vi "Main.vi"() -> ()   [LabVIEW 2013] (continued)
                # "Selection Order No"
                n1184 = Concatenate Strings(".*_" ("string"), w1862, "_" ("string")) -> (w1860:string)
              }
            }
            n1185 = call "Folder - Subtract Number of Months.vi"("- # of Months"=0, "YYYYmm"="201301", "Folder"=w1812) -> (">= Range (Folder\\YYYY\\mm)"=w1810:path[])  [unwired: 6 in, 2 out]
            n1186 = for {
              tunnel: [w1828] -> w1809 mode=concatenating
              tunnel: w1810 -> [w1827] mode=indexing
              n1187 = List Folder(path=w1827) -> (filenames=w1828:string[])  [unwired: 3 in, 3 out]
            }
            n1188 = for {
              tunnel: w1823 -> [w1852] mode=indexing
              tunnel: w1822 -> [w1854]
              tunnel: [w1853] -> w1821 mode=indexing
              n1189 = Concatenate Strings(w1854, w1852) -> (w1853:string)
            }
            n1190 = for {
              tunnel: w1821 -> [w1841] mode=indexing
              tunnel: w1809 -> [w1840]
              shift-right: [w1839] -> w1819
              shift-left: string[] [] -> [w1838]
              n1191 = for {
                tunnel: w1841 -> [w1843]
                tunnel: w1840 -> [w1844] mode=indexing
                shift-right: [w1846] -> w1839
                shift-left: w1838 -> [w1845]
                n1192 = Match Pattern(string=w1844, regular expression=w1843) -> (offset past match=w1842:i32)  [unwired: 1 in, 3 out]
                n1193 = Greater Or Equal To 0?(x=w1842) -> (x >= 0?=w1847:bool)
                n1194 = case shown="True" w1847 {
                  tunnel: w1844 -> [_ w1849]
                  tunnel: [w1848 w1851] -> w1846
                  tunnel: w1845 -> [w1848 w1850]
                  frame False {
                  }
                  frame True {
                    n1195 = Build Array (concatenate)(w1850, w1849) -> (w1851:string[])
                  }
                }
              }
            }
            "List Of Files From Selected Reports" <- w1819
            n1196 = for {
              tunnel: w1819 -> [w1837] mode=indexing
              tunnel: [w1836] -> w1818 mode=indexing
              tunnel: [w1833] -> w1817 mode=indexing
              tunnel: [w1829] -> w1814 mode=indexing
              w1834 = "_" ("regular expression")
              n1197 = Match Pattern(string=w1837, regular expression=w1834) -> (before substring=w1836:string, after substring=w1835:string)  [unwired: 1 in, 2 out]
              n1198 = Match Pattern(string=w1835, regular expression=w1834) -> (before substring=w1833:string, after substring=w1832:string)  [unwired: 1 in, 2 out]
              n1199 = Match Pattern(string=w1832, regular expression="\\.") -> (before substring=w1830:string)  [unwired: 1 in, 3 out]
              n1200 = call "String - Convert String Only TimeStamp.vi"("YYYYmmdd_HHMMSS"=w1830) -> ("YYYY-mm-dd HH:MM:SS"=w1829:string)  [unwired: 10 in]
            }
            n1201 = Build Array(w1814, w1818, w1817) -> (w1816:string[][])
            n1202 = Transpose 2D Array(2D array=w1816) -> (transposed array=w1815:string[][])
            n1203 = property on="Report List" class="MCListbox (strict)"("ItemNames"=w1815, "TopLeft"=T34 {"Row"=0, "Column"=0} ("Top Left Visible Cell"), "Value"=-1 ("Report List")) -> ()  [unwired: 2 in, 2 out]
          }
          frame True {
            w1874 = 86400.0  # 60s x 60min x 24hr
            w1879 = "[CreatedOn] >= '<A>' AND [CreatedOn] <= '<B>'"  # AND <AND_CONDITION>
            # "Move to Top"
            # "To cater for Time stored in DB but ignored in Date Control\ni.e. 2014/10/04 13:00 will be 2014/10/04 without the time\nby added 1day, it will now be 2014/10/05 which will take care of\nany TIME during the day of 2014/10/04 stored in DB"
            # "Use DB"
            n1204 = String Length(string=w1889) -> (length=w1891:i32)
            n1205 = Greater Than 0?(x=w1891) -> (x > 0?=w1890:bool)
            n1206 = case shown="True" w1890 {
              tunnel: w1889 -> [w1893 _]
              tunnel: [w1892 w1896] -> w1888
              tunnel: w1887 -> [_ w1895]
              frame True {
                # "Select by TransactionNo"
                n1207 = Bundle("TransactionNo", "Selection Transaction No"=w1893) -> (w1892:cluster{string, "Selection Transaction No":T5})  [unwired: 1 in]
              }
              frame False {
                # "Select by OrderNo"
                n1208 = Bundle("OrderNo", "Selection Order No"=w1895) -> (w1896:cluster{string, "Selection Order No":T5})  [unwired: 1 in]
              }
            }
            n1209 = property on="Date End" class="AbsTime (strict)"() -> ("Value"=w1875:timestamp)  [unwired: 2 in, 2 out]
            n1210 = property on="Date Start" class="AbsTime (strict)"() -> ("Value"=w1877:timestamp)  [unwired: 2 in, 2 out]
            n1211 = global read "Global SRTRS.vi" "Date Format"() -> (w1878:string)
            n1212 = Add(x=w1875, y=w1874) -> (x+y=w1873:timestamp)
            n1213 = Format Date/Time String(time format string (%c)=w1878, seconds (now)=w1877) -> (date/time string=w1883:string)  [unwired: 1 in]
            n1214 = Format Date/Time String(time format string (%c)=w1878, seconds (now)=w1873) -> (date/time string=w1884:string)  [unwired: 1 in]
            n1215 = Search and Replace String(input string=w1879, search string="<A>", replace string=w1883) -> (result string=w1881:string)  [unwired: 5 in, 3 out]
            n1216 = Search and Replace String(input string=w1881, search string="<B>", replace string=w1884) -> (result string=w1876:string)  [unwired: 5 in, 3 out]
            n1217 = call "DB - [Execute].[ReportList].vi"(2:DB_-_Execute_ReportList_Enum."SELECT [TransactionNo],* OR [OrderNo],*", "AND <AND_CONDITION>"=w1876, "Search Cluster"=w1888) -> ("data"=w1872:string[][], "SUMMARY"=w1885:errorcluster)  [unwired: 9 in, 2 out]
            n1218 = local write "DB"(w1885) -> ()
            n1219 = property on="Report List" class="MCListbox (strict)"("ItemNames"=w1872, "TopLeft"=T34 {"Row"=0, "Column"=0} ("Top Left Visible Cell")) -> ()  [unwired: 2 in, 2 out]
            n1220 = Array Size(array=w1872) -> (size(s)=w1871:i32[])
            n1221 = Index Array(array=w1871, index=0) -> (element=w1869:i32)
            n1222 = Greater Than 0?(x=w1869) -> (x > 0?=w1868:bool)
            n1223 = Select(t=T30."Enabled" ("Disabled"), s=w1868, f=T30."Disabled and Grayed Out" ("Disabled")) -> (s? t:f=w1866:T30)
            n1224 = property on="Report Open" class="Bool"("DisabledEnum"=w1866) -> ()  [unwired: 2 in, 2 out]
          }
        }
      }
      event "Report List": Mouse Up {
        # "Mouse UP has best result for sorting Col"
        n1225 = event-data() -> ("CtlRef"=w1900:refnum<vi>)  [unwired: 1 in, 7 out]
        n1226 = control-ref of="Sort Order"() -> (w1899:refnum<vi>)
        n1227 = call "MCListbox Event - Sort Table.vi"("Clicked Color"=u32 16777216, "Sort Order Boolean Ref"=w1899, "MCListBox Ref"=w1900) -> ()  [unwired: 8 in, 1 out]
      }
      event Value Change {
        n1228 = event-data() -> ()  [unwired: 1 in, 6 out]
        n1229 = local read "DB - Report"() -> (w1901:bool)
        n1230 = case shown="True" w1901 {
          frame False {
          }
          frame True {
            n1231 = property on="Selection Order No" class="CmbBox (strict)"() -> ("Value"=w1907:T5)  [unwired: 2 in, 2 out]
            n1232 = property on="Selection Transaction No" class="CmbBox (strict)"() -> ("Value"=w1908:T5)  [unwired: 2 in, 2 out]
            n1233 = call <vilib>:"Trim Whitespace.vi"("string"=w1907) -> ("trimmed string"=w1905:string)  [unwired: 1 in]
            n1234 = call <vilib>:"Trim Whitespace.vi"("string"=w1908) -> ("trimmed string"=w1906:string)  [unwired: 1 in]
            n1235 = String Length(string=w1905) -> (length=w1903:i32)
            n1236 = String Length(string=w1906) -> (length=w1904:i32)
            n1237 = Add(x=w1904, y=w1903) -> (x+y=w1902:i32)
            n1238 = disable-structure shown="Disabled" {
              disable-tunnel: w1902 -> [w1913 _]
              frame Disabled {
                n1239 = Greater Than 0?(x=w1913) -> (x > 0?=w1912:bool)
                n1240 = Select(t=T30."Enabled" ("Disabled"), s=w1912, f=T30."Disabled and Grayed Out" ("Disabled")) -> (s? t:f=w1909:T30)
                n1241 = property on="Report Execute Search" class="Bool"("DisabledEnum"=w1909) -> ()  [unwired: 2 in, 2 out]
              }
              frame Enabled {
              }
            }
          }
        }
      }
      event "FTP File List": Mouse Up {
        # "Mouse Up seems to work BEST for Sorting"
        n1242 = event-data() -> ("CtlRef"=w1914:refnum<vi>)  [unwired: 1 in, 7 out]
        n1243 = control-ref of="Ascending"() -> (w1915:refnum<vi>)
        n1244 = call "MCListbox Event - Sort Table.vi"("Clicked Color"=u32 16777216, "Sort Order Boolean Ref"=w1915, "MCListBox Ref"=w1914) -> ()  [unwired: 8 in, 1 out]
      }
      event "FTP File List": Value Change {
        n1245 = event-data() -> ("NewVal"=w1919:i32)  [unwired: 1 in, 5 out]
        n1246 = global read "Global SRTRS.vi" "[RawDataReport]"() -> (w1917:bool)
        n1247 = Greater Or Equal To 0?(x=w1919) -> (x >= 0?=w1918:bool)
        n1248 = case shown="True" w1917 {
          tunnel: w1918 -> [_ w1923]
          frame False {
          }
          frame True {
            n1249 = Select(t=T30."Enabled" ("Disabled"), s=w1923, f=T30."Disabled and Grayed Out" ("Disabled")) -> (s? t:f=w1922:T30)
            n1250 = property on="cRIO FTP Copy" class="Bool"("DisabledEnum"=w1922) -> ()  [unwired: 2 in, 2 out]
          }
        }
      }
      event "cRIO  Search": Value Change {
        (unwired) "c:\\ni-rt\\LabVIEW Data\\SRTRS4070\\Data\\"
        w1939 = "\\" ("string")
        # "c:\\ni-rt\\LabVIEW Data\\SRTRS4070\\Data\\2014\\04\\"
        # "FTP to cRIO to look for raw data files"
        n1251 = event-data() -> ()  [unwired: 1 in, 6 out]
        n1252 = local read "cRIO IP"() -> (w1946:string)
        n1253 = Format Into String(format string="%02d", "FTP Month") -> (resulting string=w1936:string)  [unwired: 2 in, 1 out]
        n1254 = Format Into String("FTP Year") -> (resulting string=w1940:string)  [unwired: 3 in, 1 out]
        n1255 = Concatenate Strings("u:\\ni-rt\\LabVIEW Data\\SRTRS4070\\Data\\", w1940, w1939, w1936, w1939) -> (w1938:string)
        n1256 = call "cRIO - FTP Module.vi"("List"=TRUE, "Copy"=FALSE, "Source Folder (on RT target)"=w1938, "IP address of remote RT target"=w1946) -> ("Error Out"=w1935:errorcluster, "Files in cRIO"=w1943:string[])  [unwired: 4 in, 2 out]
        n1257 = case shown="No Error" w1935 {
          tunnel: w1943 -> [w1956 _]
          tunnel: [w1951 _] -> w1931
          frame No Error {
            n1258 = String To Path(string=w1956) -> (path=w1955:path[])
            n1259 = for {
              tunnel: w1955 -> [w1964] mode=indexing
              tunnel: [w1958] -> w1954 mode=indexing
              tunnel: [w1957] -> w1953 mode=indexing
              n1260 = Strip Path(path=w1964) -> (name=w1963:string)  [unwired: 1 out]
              n1261 = Match Pattern "Transaction No."(string=w1963, regular expression="_") -> (before substring=w1957:string, after substring=w1962:string)  [unwired: 1 in, 2 out]
              n1262 = Match Pattern "Time Stamp"(string=w1962, regular expression=".dat") -> (before substring=w1959:string)  [unwired: 1 in, 3 out]
              n1263 = call "String - Convert String Only TimeStamp.vi"("YYYYmmdd_HHMMSS"=w1959) -> ("YYYY-mm-dd HH:MM:SS"=w1958:string)  [unwired: 10 in]
            }
            n1264 = Build Array(w1954, w1953) -> (w1952:string[][])
            n1265 = Transpose 2D Array(2D array=w1952) -> (transposed array=w1951:string[][])
            "Files in cRIO" <- w1956
          }
          frame Error {
          }
        }
        n1266 = Array Size(array=w1931) -> (size(s)=w1930:i32[])
        n1267 = Index Array(array=w1930) -> (element=w1924:i32)  [unwired: 1 in]
        n1268 = property on="FTP File List" class="MCListbox (strict)"("ItemNames"=w1931, "TopLeft"=T34 {"Row"=0, "Column"=0} ("Top Left Visible Cell"), "Value"=-1 ("Report List")) -> ()  [unwired: 2 in, 2 out]
        n1269 = Format Into String(w1924) -> (resulting string=w1929:string)  [unwired: 3 in, 1 out]
        n1270 = case shown="0" w1924 {
          frame 1, Default {
          }
          frame 0 {
            n1271 = call "Msgbox - Message Handler.vi"("Short Description (When DB Not Available)"="Raw Data Not Found", "Description (When DB Not Available)"="No raw data files for the given criteria", "<.?....> Message Code"="<E 403>") -> ("MHandler Error"=w1947:errorcluster)  [unwired: 6 in, 2 out]
            n1272 = local write "MHandler"(w1947) -> ()
          }
        }
        n1273 = Concatenate Strings("{cRIO Search} " ("string"), w1929, " file(s) found." ("string")) -> (w1925:string)
        n1274 = call "Queue - EnQueue to MessageQ.vi"("<NoD> Don't Display to UI"=TRUE, "Message"=w1925) -> ()  [unwired: 9 in, 1 out]
      }
      event "cRIO FTP Copy": Value Change {
        n1275 = event-data() -> ()  [unwired: 1 in, 6 out]
        n1276 = local read "FTP File List"() -> (w1965:i32)
        n1277 = case shown="0, Default" w1965 {
          selector: w1965 -> [w1974 _]
          frame 0, Default {
            # "1076_20150109_130402.dat"
            # "1076_2015-01-09_13:04:02.dat"
            # "1076_2015-01-09  13:04:02.dat"
            # "2015-01-09  13:04:02"
            # "Items may be sorted, so \ndifferent order in Files in cRIO array"
            # "1008_20141120_091147.dat"
            # "0090300742_20140822_114859.dat"
            # "Valid Selection"
            n1278 = property on="FTP File List" class="MCListbox (strict)"() -> ("ItemNames"=w1982:string[][])  [unwired: 2 in, 2 out]
            n1279 = Index Array(array=w1982, index (row)=w1974) -> (element=w1981:string[])  [unwired: 1 in]
            n1280 = Index Array(array=w1981) -> (element #1=w1978:string, element #2=w1980:string)  [unwired: 2 in]
            n1281 = local read "Files in cRIO"() -> (w1976:string[])
            n1282 = Concatenate Strings(w1980, "_", w1978, ".dat" ("string")) -> (w1967:string)
            n1283 = Search and Replace String(replace all?=TRUE ("replace all? (F)"), input string=w1967, search string="  ", replace string="_" ("replace string (\"\")")) -> (result string=w1971:string)  [unwired: 4 in, 3 out]
            n1284 = Search and Replace String(replace all?=TRUE ("replace all? (F)"), input string=w1971, search string="[-:]") -> (result string=w1966:string)  [unwired: 5 in, 3 out]
            n1285 = for {
              tunnel: w1976 -> [w2006] mode=indexing
              tunnel: w1966 -> [w2009]
              tunnel: [w2006] -> w1975
              stop <- w2007 stop-if-true
              n1286 = Match Pattern(string=w2006, regular expression=w2009) -> (offset past match=w2008:i32)  [unwired: 1 in, 3 out]
              n1287 = Greater Or Equal To 0?(x=w2008) -> (x >= 0?=w2007:bool)
            }
            "Source File Path (on RT Target)" <- w1975
            n1288 = local read "Data"() -> (w1992:path)
            n1289 = String To Path(string=w1975) -> (path=w2000:path)
            n1290 = local read "cRIO IP"() -> (w2005:string)
            n1291 = Strip Path(path=w2000) -> (name=w1999:string)  [unwired: 1 out]
            n1292 = Match Pattern(string=w1999, regular expression="_") -> (after substring=w1990:string)  [unwired: 1 in, 3 out]
            n1293 = String Subset(string=w1990, length (rest)=4 ("length (rest)")) -> (substring=w1996:string)  [unwired: 1 in]
            n1294 = String Subset(string=w1990, offset (0)=4, length (rest)=2 ("length (rest)")) -> (substring=w1993:string)
            n1295 = Concatenate Strings(w1996, "\\" ("string"), w1993) -> (w1991:string)
            n1296 = Build Path(base path=w1992, name or relative path=w1991) -> (appended path=w1984:path)
            "Destination Folder (on Local Host)" <- w1984
            n1297 = call "cRIO - FTP Module.vi"("List"=FALSE, "Destination Folder (on local host)"=w1984, "Copy"=TRUE, "Source File Path (on RT Target)"=w1975, "IP address of remote RT target"=w2005) -> ("Error Out"=w2002:errorcluster, "Destination File Path (on local host)"=w2001:path)  [unwired: 3 in, 2 out]
            "Destination File Path (on local host)" <- w2001
            "cRIO FTP Module (Error Out)" <- w2002
            n1298 = case shown="Error" w2002 {
              selector: w2002 -> [_ w2032]
              tunnel: w2001 -> [w2020 _]
              tunnel: [w2018 "Raw Data Not Retrieved" ("Short Description (When DB Not Available)")] -> w1988
              tunnel: [w2017 "Raw data not retrieved to the folder " ("Short Description (When DB Not Available)")] -> w1987
              tunnel: [w2016 "<E 407>" ("Short Description (When DB Not Available)")] -> w1986
              tunnel: [w2010 w2027] -> w1985
              tunnel: w1984 -> [w2011 w2028]
              frame No Error {
                # "Use Server Folder if blank"
                n1299 = call <vilib>:"Check if File or Folder Exists.vi"("path"=w2020) -> ("file or folder exists?"=w2019:bool, "dup path"=w2012:path)  [unwired: 8 in, 1 out]
                n1300 = Path To String(path=w2012) -> (string=w2013:string)
                n1301 = Path To String(path=w2011) -> (string=w2015:string)
                n1302 = Empty String/Path?(string/path=w2013) -> (empty?=w2014:bool)
                n1303 = Select(t=w2015, s=w2014, f=w2013) -> (s? t:f=w2010:string)
                n1304 = case shown="False" w2019 {
                  tunnel: ["Raw Data Not Retrieved" ("Short Description (When DB Not Available)") "Raw Data Retrieved" ("Short Description (When DB Not Available)")] -> w2018
                  tunnel: ["Raw data not retrieved to the folder " ("Short Description (When DB Not Available)") "Raw data retrieved to the folder " ("Short Description (When DB Not Available)")] -> w2017
                  tunnel: ["<E 407>" ("Short Description (When DB Not Available)") "<I 404>" ("Short Description (When DB Not Available)")] -> w2016
                  frame False {
                  }
                  frame True {
                  }
                }
              }
              frame Error {
                n1305 = Unbundle By Name(w2032) -> ()  [unwired: 1 out]
                n1306 = Path To String(path=w2028) -> (string=w2027:string)
              }
            }
            n1307 = call "Msgbox - Message Handler.vi"("Short Description (When DB Not Available)"=w1988, "Description (When DB Not Available)"=w1987, "Post-Description"=w1985, "<.?....> Message Code"=w1986) -> ("MHandler Error"=w1983:errorcluster)  [unwired: 5 in, 2 out]
            n1308 = local write "MHandler"(w1983) -> ()
          }
          frame -1 {
            # "None selected"
          }
        }
      }
      event "Report Open": Value Change; "Report List": Double Click {
        # "cmd  /c  start acrord32.exe \"c:\\temp\\SRTRS4070\\Reports\\YYYY\\mm\\0090300205_123456002_20131223_164339.pdf\""
        # "Report File\n<Transaction Number>_<Order Number>_<Date>_<Time>.pdf"
        n1309 = event-data() -> ("CtlRef"=w2036:refnum<vi>)  [unwired: 1 in, 3 out]
        n1310 = property class="Ctl"(reference=w2036) -> (reference out=w2033:refnum<vi>, "Label.Text"=w2035:string)  [unwired: 1 in, 1 out]
        n1311 = case shown="\"Report List\"" w2035 {
          tunnel: [TRUE w2107] -> w2034
          tunnel: w2033 -> [_ _]
          frame "False", Default {
          }
          frame "Report List" {
            n1312 = local read "Report List"() -> (w2106:i32)
            n1313 = Greater Or Equal To 0?(x=w2106) -> (x >= 0?=w2107:bool)
          }
        }
        n1314 = case shown="True" w2034 {
          frame False {
          }
          frame True {
            w2046 = "\"" ("string")
            n1315 = local read "DB - Report"() -> (w2039:bool)
            n1316 = case shown="True" w2039 {
              tunnel: [w2057 w2077] -> w2045
              frame False {
                # "YYYY\\mm"
                # "<Transaction Number>"
                n1317 = local read "List Of Files From Selected Reports"() -> (w2066:string[])
                n1318 = local read "Report List"() -> (w2065:i32)
                n1319 = Index Array(array=w2066, index=w2065) -> (element=w2059:string)
                n1320 = Match Pattern(string=w2059, regular expression="_") -> (after substring=w2063:string)  [unwired: 1 in, 3 out]
                n1321 = local read "Reports"() -> (w2056:path)
                n1322 = Match Pattern(string=w2063, regular expression="_") -> (after substring=w2055:string)  [unwired: 1 in, 3 out]
                n1323 = String Subset(string=w2055, length (rest)=4 ("length (rest)")) -> (substring=w2051:string)  [unwired: 1 in]
                n1324 = String Subset(string=w2055, offset (0)=4, length (rest)=2 ("length (rest)")) -> (substring=w2052:string)
                n1325 = Concatenate Strings(w2051, "\\" ("string"), w2052) -> (w2049:string)
                n1326 = Build Path(base path=w2056, name or relative path=w2049) -> (appended path=w2064:path)
                n1327 = Build Path(base path=w2064, name or relative path=w2059) -> (appended path=w2058:path)
                n1328 = Path To String(path=w2058) -> (string=w2057:string)
              }
              frame True {
                w2076 = 6  # [LayoutId]
                (unwired) string[] ["Date and Time", "Transaction No.", "Transaction\n Run No.", "Order No.", "Number \nof Orders", "Report \nRun No.", "Layout ID"]  # 2014-11-11 08:55 Column Header Strings[]
                w2081 = 1  # [ReportFileName]
                w2082 = 0  # [ReportFilePath]
                w2083 = 0 ("index (row)")
                w2096 = "[TransactionNo] = '<A>' \nAND [TransactionRunNo] = '<B>' \nAND [OrderNo] = '<C>' \nAND [ReportRunNo] = '<D>'\nAND [LayoutId] <E>"  # AND <AND_CONDITION>
                w2097 = 5  # [ReportRunNo]
                w2098 = 3  # [OrderNo]
                w2099 = 2  # [TransactionRunNo]
                w2100 = 1  # [TransactionNo]
                # "Legacy : Caters for no LayoutId"
                # "Use DB"
                n1329 = property on="Report List" class="MCListbox (strict)"() -> ("Value"=w2102:i32)  [unwired: 2 in, 2 out]
                n1330 = property on="Report List" class="MCListbox (strict)"() -> ("ItemNames"=w2103:string[][])  [unwired: 2 in, 2 out]
                n1331 = Index Array(array=w2103, index (row)=w2102) -> (element=w2101:string[])  [unwired: 1 in]
                n1332 = Index Array(array=w2101, index #1=w2100, index #2=w2099, index #3=w2098, index #4=w2097, index #5=w2076) -> (element #1=w2088:string, element #2=w2087:string, element #3=w2086:string, element #4=w2085:string, element #5=w2068:string)
                n1333 = Search and Replace String(input string=w2096, search string="<A>", replace string=w2088) -> (result string=w2092:string)  [unwired: 5 in, 3 out]
                n1334 = Empty String/Path?(string/path=w2068) -> (empty?=w2072:bool)
                n1335 = Format Into String(format string=" = '%s'", w2068) -> (resulting string=w2067:string)  [unwired: 2 in, 1 out]
                n1336 = Search and Replace String(input string=w2092, search string="<B>", replace string=w2087) -> (result string=w2095:string)  [unwired: 5 in, 3 out]
                n1337 = Search and Replace String(input string=w2095, search string="<C>", replace string=w2086) -> (result string=w2094:string)  [unwired: 5 in, 3 out]
                n1338 = Select(t="is NULL", s=w2072, f=w2067) -> (s? t:f=w2070:string)
                n1339 = Search and Replace String(input string=w2094, search string="<D>", replace string=w2085) -> (result string=w2075:string)  [unwired: 5 in, 3 out]
                n1340 = Search and Replace String(input string=w2075, search string="<E>", replace string=w2070) -> (result string=w2073:string)  [unwired: 5 in, 3 out]
                n1341 = call "DB - [Execute].[ReportList].vi"(2:DB_-_Execute_ReportList_Enum."SELECT [ReportFileName]", "AND <AND_CONDITION>"=w2073) -> ("data"=w2084:string[][])  [unwired: 10 in, 3 out]
                n1342 = Index Array(array=w2084, index (row) #1=w2083, index (col) #1=w2082, index (row) #2=w2083, index (col) #2=w2081) -> (element #1=w2080:string, element #2=w2078:string)
                n1343 = Concatenate Strings(w2080, "\\" ("string"), w2078) -> (w2077:string)
              }
            }
            n1344 = Concatenate Strings(w2046, w2045, w2046) -> (w2041:string)
            n1345 = Concatenate Strings("cmd  /c  start acrord32.exe " ("string"), w2041) -> (w2043:string)
            n1346 = call <vilib>:"System Exec.vi"("run minimized? (F)"=TRUE, "wait until completion? (T)"=FALSE, "command line"=w2043) -> ()  [unwired: 5 in, 4 out]
            n1347 = Concatenate Strings("{OPEN REPORT} Clicked By User. " ("string"), w2041, " is selected." ("string")) -> (w2038:string)
            n1348 = call "Queue - EnQueue to MessageQ.vi"("<NoD> Don't Display to UI"=TRUE, "Message"=w2038) -> ()  [unwired: 9 in, 1 out]
          }
        }
      }
      event "Report List": Value Change {
        n1349 = event-data() -> ("NewVal"=w2108:i32)  [unwired: 1 in, 5 out]
        n1350 = case shown="0, Default" w2108 {
          frame 0, Default {
            n1351 = property on="Report Open" class="Bool"("DisabledEnum"=T30."Enabled" ("Disabled")) -> ()  [unwired: 2 in, 2 out]
          }
          frame -1 {
          }
        }
      }
      event "Report Generate": Value Change {
        # "This will be '0' if\nReport is AutoGenerated"
        # "USER Clicks on Generate Report Button"
        n1352 = event-data() -> ()  [unwired: 1 in, 6 out]
        n1353 = local read "ReportList Cluster"() -> (w2124:T18)
        n1354 = Bundle By Name(cluster=w2124, "[IsManual]"="1") -> (w2125:T18)
        n1355 = local write "Logon (Report Buffer)"(T21 {"PlantID"="", "SystemID"="", "UserID"="", "DomainID"="", "LanguageID"="", "StationID"=""} ("Logon (Report Buffer)")) -> ()
        n1356 = local write "ReportList Cluster"(w2125) -> ()
        n1357 = local read "Raw Data File (Report Tab)"() -> (w2110:path)
        n1358 = global read "Global SRTRS.vi" "DB Available"() -> (w2111:bool)
        n1359 = Strip Path(path=w2110) -> (name=w2122:string)  [unwired: 1 out]
        n1360 = case shown="False" w2111 {
          tunnel: [TRUE ("[RawDataReport]") w2128] -> w2118
          frame False {
          }
          frame True {
            # "Check only if DB Available"
            n1361 = global read "Global SRTRS.vi" "[RawDataReport]"() -> (w2128:bool)
          }
        }
        n1362 = Match Pattern(string=w2122, regular expression=".dat") -> (offset past match=w2120:i32)  [unwired: 1 in, 3 out]
        n1363 = call <vilib>:"Check if File or Folder Exists.vi"("path"=w2110) -> ("file or folder exists?"=w2116:bool)  [unwired: 8 in, 2 out]
        n1364 = Greater Or Equal To 0?(x=w2120) -> (x >= 0?=w2117:bool)
        n1365 = Compound Arithmetic op=AND(w2118, w2117, w2116) -> (w2119:bool)
        n1366 = case shown="True" w2119 {
          tunnel: w2122 -> [_ w2147]
          tunnel: w2118 -> [w2139 _]
          tunnel: w2117 -> [w2138 _]
          tunnel: w2116 -> [w2135 _]
          tunnel: [w2133 "File Exists."] -> w2113
          tunnel: w2110 -> [_ w2144]
          frame False {
            n1367 = case shown="False" w2139 {
              tunnel: ["You have no access. " _] -> w2137
              frame False {
              }
              frame True {
              }
            }
            n1368 = case shown="False" w2138 {
              tunnel: ["Not a .dat file. " _] -> w2136
              frame False {
              }
              frame True {
              }
            }
            n1369 = case shown="False" w2135 {
              tunnel: ["File/Folder does not exists. " _] -> w2134
              frame False {
              }
              frame True {
              }
            }
            n1370 = Concatenate Strings(w2137, w2136, w2134) -> (w2133:string)
            n1371 = call "Msgbox - Message Handler.vi"("Short Description (When DB Not Available)"="Report Generate Failed", "Description (When DB Not Available)"="Please check output set and file server availability and Retry", "<.?....> Message Code"="<E 406>") -> ("MHandler Error"=w2132:errorcluster)  [unwired: 6 in, 2 out]
            n1372 = local write "MHandler"(w2132) -> ()
          }
          frame True {
            n1373 = global read "Global SRTRS.vi" "DB Available"() -> (w2145:bool)
            n1374 = case shown="True" w2145 {
              tunnel: w2147 -> [_ w2164]
              tunnel: w2144 -> [w2152 _]
              tunnel: [w2148 w2153] -> w2143
              frame False {
                n1375 = Strip Path(path=w2152) -> (name=w2151:string)  [unwired: 1 out]
                n1376 = Match Pattern "TransactionNo"(string=w2151, regular expression="_") -> (before substring=w2149:string)  [unwired: 1 in, 3 out]
                n1377 = Empty String/Path?(string/path=w2149) -> (empty?=w2148:bool)
              }
              frame True {
                # "Only check if DB Available"
                n1378 = call "DB - [Execute].[Transaction].vi"("DB.Schema.Table"="SRTRS.Execute.TransactionResult", "DB - Execute Transaction"=DB_-_Execute_Transaction_Enum."SELECT [TransactionNo],[TransactionRunNo]", "[RawDataFileName]"=w2164) -> ("Transaction"=w2160:T19, "SUMMARY"=w2163:errorcluster)  [unwired: 13 in, 2 out]
                n1379 = local write "DB"(w2163) -> ()
                n1380 = local write "Transaction (Report Buffer)"(w2160) -> ()
                n1381 = Unbundle By Name(w2160) -> ("TransactionNo"=w2158:string, "TransactionRunNo"=w2159:string)
                n1382 = Unbundle By Name(w2163) -> ("status"=w2154:bool)
                n1383 = Empty String/Path?(string/path=w2158) -> (empty?=w2157:bool)
                n1384 = Empty String/Path?(string/path=w2159) -> (empty?=w2156:bool)
                n1385 = Or(x=w2157, y=w2156) -> (x .or. y?=w2155:bool)
                n1386 = Or(x=w2155, y=w2154) -> (x .or. y?=w2153:bool)
              }
            }
            n1387 = case shown="False" w2143 {
              frame False {
                # "Proceed to Generate Report"
                n1388 = property on="Report Generate Toggle" class="Bool (strict)"() -> ("Value"=w2166:bool)  [unwired: 2 in, 2 out]
                n1389 = Not(x=w2166) -> (.not. x?=w2165:bool)
                n1390 = property on="Report Generate Toggle" class="Bool (strict)"("Val(Sgnl)"=w2165) -> ()  [unwired: 2 in, 2 out]
              }
              frame True {
                # "DB Error OR Either TxNo or TxRunNo is missing"
                n1391 = call "Msgbox - Message Handler.vi"("Short Description (When DB Not Available)"="Report Generation Fail", "Description (When DB Not Available)"="Please check output set availability and Retry.", "<.?....> Message Code"="<E 406>") -> ("MHandler Error"=w2167:errorcluster)  [unwired: 6 in, 2 out]
                n1392 = local write "MHandler"(w2167) -> ()
              }
            }
          }
        }
        n1393 = Concatenate Strings("{Generate Report} ", w2113) -> (w2112:string)
        n1394 = call "Queue - EnQueue to MessageQ.vi"("<NoD> Don't Display to UI"=TRUE, "Message"=w2112) -> ()  [unwired: 9 in, 1 out]
      }
      event "Report Generate Toggle": Value Change {
        # "Phase 2 Report File\n[TransactionNo]_[OrderNo]_[NoOfOrders][ReportRunNo].xls"
        # "Report File Phase 2\n<Transaction Number>_<Order Number>_<No Of Orders><ReportRunNumber>.xls"
        # "Phase 1 Report File\n<Transaction Number>_<Order Number>_<Date>_<Time>.xls"
        # "Total Columns including Key"
        # "Multiple Order Numbers"
        # "Setup Folder has no year"
        # "Report File\n<Transaction Number>_<Order Number>_<Date>_<Time>.xls"
        # "Raw Data File\n<Transaction Number>_<Date>_<Time>.dat"
        # "Setup File\n<Transaction Number>_<Date>_<Time>.stp"
        # "Date and Time may be different. Setup File is created before Raw Data File."
        # "Create Report File from Raw Data File and DB OR Setup File\n[IsManual] determines if it was auto generated or from User initiated"
        n1395 = event-data() -> ()  [unwired: 1 in, 6 out]
        n1396 = case shown="True" "DB - Report" {
          tunnel: w2213 -> [w2432 _]
          tunnel: w2212 -> [w2422 _]
          tunnel: [w2418 w2500] -> w2210
          tunnel: [w2415 w2488] -> w2173
          tunnel: [w2414 w2554] -> w2205
          tunnel: [w2400 w2535] -> w2197
          tunnel: [w2395 w2516] -> w2195
          tunnel: [w2394 w2515] -> w2194
          frame False {
            (unwired) string[][] [["No", "1", "2"], ["Order No", "101", "102"], ["Customer Name", "Cust101", "Cust102"]]
            w2429 = 1  # # of Cols
            # "Sequence Number,  1,2,3,\nRamp Rate,                60,60,30,\nTarget Temperature,32,36,26,\nHold Time,                 00:01,00:02,00:00,\nAdditional WPS,\nRev.,\nName,Temperature Controller,Temperature Module (NI),Temperature Module (NI)\nModel,ET-3504,NI-9211,NI-9211\nSerial No.,E123-02,12F0001,12F0002\nLast Cal. Date,22-12-2013,01-01-2014,02-02-2014\nNext Cal. Due Date,22-12-2015,30-01-2015,28-02-2015\nEquipment ID,ET-3504 02,NI-9211 01,NI-9211 02\nNotice Period,30,30,60\nCal. Required,-1,-1,-1\nWPS/Ref,WPS5\nRev,3\nHold Temperature,36\nWPS Details Temperature Units,°C\nHold Time (HH:MM),00:02\nInactive,F\nFurnace Serial No,A1234A1\nLast Calibration Date,22-12-2013\nNext Calibration Due Date,22-12-2015\nChannel to Probe Mapping,1,2,3,4,5,6,7,8,9,10,11,12,13,14,15,16"
            # "1st Column is Label, so must minus 1"
            # "No, 1 ,2\nOrder No, 101, 102\nCustomer Name, Cust101, Cust102"
            # "String was stored as , seperated"
            # "Changed to TAB"
            # "Look 3 mths ahead"
            # "_<Date>_<Time>.dat"
            # "Easier to maintain code if on seperate loop"
            # "Key1 = value1, value2\nKey2 = value1a, value2a"
            # "Setup File"
            # "There should only be one found"
            # "<Transaction Number>"
            # "USE stp, wps, jpg Files and for REPORT"
            n1397 = local read "Raw Data File (Report Tab)"() -> (w2399:path)
            n1398 = Array Subset "Ignore Part Details\nTake the Other 3 MCListbox"(array=w2432, index=1) -> (w2423:refnum<vi>[])  [unwired: 1 in]
            n1399 = Index Array(array=w2432, index=0) -> (element=w2420:refnum<vi>)
            n1400 = Strip Path(path=w2399) -> (name=w2440:string)  [unwired: 1 out]
            n1401 = Build Array (concatenate)(w2423, w2422) -> (w2421:refnum<vi>[])
            n1402 = Match Pattern(string=w2440, regular expression="_") -> (before substring=w2400:string, after substring=w2439:string)  [unwired: 1 in, 2 out]
            n1403 = local read "Setup"() -> (w2408:path)
            n1404 = Concatenate Strings(w2400, "_*.stp" ("string")) -> (w2435:string)
            n1405 = Match Pattern(string=w2439, regular expression="_") -> (before substring=w2413:string)  [unwired: 1 in, 3 out]
            n1406 = local read "Layout ID"() -> (w2392:string)
            n1407 = String Subset(string=w2413, length (rest)=4 ("length (rest)")) -> (substring=w2410:string)  [unwired: 1 in]
            n1408 = String Subset(string=w2413, offset (0)=4, length (rest)=2 ("length (rest)")) -> (substring=w2409:string)
            n1409 = Build Array(w2392) -> (w2394:string[])
            n1410 = local read "Template File"() -> (w2393:path)
            n1411 = Concatenate Strings(w2410, w2409) -> (w2406:string)
            "YYYYmm" <- w2406
            n1412 = call "Folder - Subtract Number of Months.vi"("- # of Months"=3, "YYYYmm"=w2406, "Folder"=w2408) -> (">= Range (Folder\\YYYY\\mm)"=w2405:path[])  [unwired: 6 in, 2 out]
            n1413 = for {
              tunnel: w2435 -> [w2466]
              tunnel: w2405 -> [w2465] mode=indexing
              tunnel: [w2464] -> w2404
              tunnel: [w2461] -> w2403
              stop <- w2462 stop-if-true
              n1414 = List Folder(path=w2465, pattern=w2466) -> (path out=w2464:path, filenames=w2463:string[])  [unwired: 2 in, 2 out]
              n1415 = for {
                tunnel: w2463 -> [w2469] mode=indexing
                tunnel: [w2467] -> w2462
                tunnel: [w2469] -> w2461
                stop <- w2467 stop-if-true
                n1416 = Empty String/Path?(string/path=w2469) -> (empty?=w2468:bool)
                n1417 = Not(x=w2468) -> (.not. x?=w2467:bool)
              }
            }
            n1418 = Build Path(base path=w2404, name or relative path=w2403) -> (appended path=w2402:path)
            n1419 = Not A Number/Path/Refnum?(number/path/refnum=w2402) -> (NaN/Path/Refnum?=w2401:bool)
            n1420 = Build Array(w2393) -> (w2395:path[])
            n1421 = case shown="True" w2401 {
              tunnel: w2400 -> [_ w2460]
              tunnel: [_ errorcluster {"status"=TRUE, "code"=-8001, "source"=" setup file (.stp) not found."} ("error in (no error)")] -> w2398
              frame False {
              }
              frame True {
                n1422 = Concatenate Strings("Transaction Number " ("string"), w2460, " setup file (.stp) not found." ("string")) -> (w2457:string)
                n1423 = One Button Dialog(message=w2457) -> ()  [unwired: 1 in, 1 out]
              }
            }
            n1424 = call <vilib>:"Open Config Data.vi"("error in (no error)"=w2398, "create file if necessary (T)"=FALSE, "configuration file path"=w2402) -> ("error out"=w2396:errorcluster, "refnum"=w2397:T59)  [unwired: 6 in, 1 out]
            n1425 = for {
              tunnel: w2421 -> [w2472] mode=indexing
              tunnel: w2397 -> [w2473]
              tunnel: w2396 -> [w2475]
              shift-right: [w2470] -> w2387
              shift-left: "" -> [w2474]
              tunnel: [w2471] -> w2416 mode=indexing
              n1426 = call "Key - Read to Spreadsheet String.vi"("error in (no error)"=w2475, "String in"=w2474, "Control in"=w2472, "ini File Ref num"=w2473) -> ("error out"=w2471:errorcluster, "String out"=w2470:string)  [unwired: 6 in]
            }
            n1427 = call "Key - Read to Spreadsheet String.vi"("error in (no error)"=w2396, "Control in"=w2420, "ini File Ref num"=w2397) -> ("error out"=w2417:errorcluster, "String out"=w2426:string)  [unwired: 7 in]
            n1428 = Merge Errors(w2417, w2416) -> (w2415:errorcluster)
            n1429 = Spreadsheet String To Array(delimiter (Tab)=",", format string="", spreadsheet string=w2426, array type (2D Dbl)=string[][] []) -> (array=w2385:string[][])
            n1430 = Spreadsheet String To Array(delimiter (Tab)=",", format string="", spreadsheet string=w2387, array type (2D Dbl)=string[][] []) -> (array=w2383:string[][])
            n1431 = Array Size(array=w2385) -> (size(s)=w2430:i32[])
            n1432 = Index Array(array=w2430, index=w2429) -> (element=w2428:i32)
            n1433 = Decrement(x=w2428) -> (x-1=w2386:i32)
            n1434 = case shown="No Error" w2396 {
              tunnel: [w2441 _] -> w2382
              tunnel: w2397 -> [w2447 _]
              frame No Error {
                # "Changed to TAB"
                n1435 = flat-sequence {
                  tunnel: w2447 -> [w2453]
                  tunnel: [w2455] -> w2446
                  frame #0 {
                    n1436 = control-ref of="Parameter Buffer"() -> (w2454:refnum<vi>)
                    n1437 = call "Key - Cluster Read.vi"("New Ctl Ref"=w2454, "Original Ctl Ref"=w2454, "Refnum in"=w2453) -> ()  [unwired: 6 in, 3 out]
                  }
                  frame #1 {
                    n1438 = local read "Parameter Buffer"() -> (w2455:T15)
                  }
                }
                n1439 = Unbundle By Name(w2446) -> ("Start Holding Time and Date"=w2445:string, "End Holding Time and Date"=w2443:string, "Start Holding Temperature"=w2451:string, "End Holding Temperature"=w2450:string)
                n1440 = Fract/Exp String To Number(string=w2451) -> (number=w2449:dbl)  [unwired: 3 in, 1 out]
                n1441 = Fract/Exp String To Number(string=w2450) -> (number=w2448:dbl)  [unwired: 3 in, 1 out]
                n1442 = call "String - Convert Str (YYYY-mm-dd HHcMMcSS) to TimeStamp.vi"("YYYY-mm-dd HH:MM:SS (String)"=w2445) -> ("time stamp"=w2444:timestamp)  [unwired: 9 in, 1 out]
                n1443 = call "String - Convert Str (YYYY-mm-dd HHcMMcSS) to TimeStamp.vi"("YYYY-mm-dd HH:MM:SS (String)"=w2443) -> ("time stamp"=w2442:timestamp)  [unwired: 9 in, 1 out]
                n1444 = local read "Info."() -> (w2452:T9)
                n1445 = call "Parameters - Update.vi"("Parameter (End Dwell Temp)"=w2448, "Parameter (Start Dwell Temp)"=w2449, "Parameter (End Dwell Time)"=w2442, "Parameter (Start Dwell Time)"=w2444, "Info."=w2452) -> ("Parameters"=w2441:string[][])  [unwired: 3 in, 3 out]
              }
              frame Error {
              }
            }
            n1446 = Build Array (concatenate)(w2383, w2382) -> (w2381:string[][])
            n1447 = call "Key - Adjust Names For Report.vi"("Parameters"=w2381) -> ("output array"=w2384:string[][])  [unwired: 10 in]
            n1448 = for {
              N: w2386 -> [_]
              tunnel: w2385 -> [w2485]
              tunnel: w2384 -> [w2481]
              tunnel: [w2482] -> w2418 mode=indexing
              tunnel: [w2486] -> w2414 mode=indexing
              i -> [w2487]
              # "All Arrays Now"
              # "List by Order Number"
              n1449 = Increment(x=w2487) -> (x+1=w2483:i32)
              n1450 = Index Array(array=w2485, index (col) #1=0 ("disabled index (col)"), index (col) #2=w2483) -> (element #1=w2476:string[], element #2=w2480:string[])  [unwired: 2 in]
              n1451 = Number To Decimal String(number=w2483) -> (decimal integer string=w2486:string)  [unwired: 1 in]
              n1452 = Build Array(w2476, w2480) -> (w2479:string[][])
              n1453 = Transpose 2D Array(2D array=w2479) -> (transposed array=w2478:string[][])
              n1454 = Build Array (concatenate)(w2478, w2481) -> (w2477:string[][])
              n1455 = Flatten To String(anything=w2477) -> (data string=w2482:string)  [unwired: 3 in, 2 out]
            }
          }
          frame True {
            w2513 = T62[] [enum."[IsTempWithinTol]", enum."[IsTimeWithinTol]"] items=["[StartRecordTime]", "[StartRecordTemp]", "[MaxRecordedTemp]", "[MaxRecordedTempTime]", "[MinRecordedTemp]", "[MinRecordedTempTime]", "[EndRecordTemp]", "[EndRecordTime]", "[RecordedMinutes]", "[StartHoldTime]", "[StartHoldTemp]", "[HoldTimeMaxTemp]", "[HoldTimeMaxTempTime]", "[HoldTimeMinTemp]", "[HoldTimeMinTempTime]", "[EndHoldTime]", "[EndHoldTemp]", "[HoldDurationMinutes]", "[TempDiffDuringHold]", "[UnitOfTemperature]", "[PerformedBy]", "[PerformedOn]", "[IsTempWithinTol]", "[IsTimeWithinTol]", "[HoldTimePercentage]", "[ProcessStatus]", "[OverallStatus]", "[SequenceStatus]", "[Parameter1]", "[Parameter2]", "[Parameter3]", "[Parameter4]", "[Parameter5]", "[Parameter6]", "[Parameter7]", "[Parameter8]", "[Parameter9]", "[Parameter10]", "[Parameter11]", "[Parameter12]", "[Result]", "[RawDataFile]", "[RawDataFilePath]", "[RawDataFileName]", "[OutputSetId]", "[SavedBy]", "[SavedOn]", "[Inactive]"]
            w2540 = T62[] [enum."[StartRecordTime]", enum."[StartRecordTemp]", enum."[MaxRecordedTemp]", enum."[MaxRecordedTempTime]", enum."[MinRecordedTemp]", enum."[MinRecordedTempTime]", enum."[EndRecordTemp]", enum."[EndRecordTime]", enum."[RecordedMinutes]", enum."[StartHoldTime]", enum."[StartHoldTemp]", enum."[HoldTimeMaxTemp]", enum."[HoldTimeMinTemp]", enum."[EndHoldTime]", enum."[EndHoldTemp]", enum."[HoldDurationMinutes]", enum."[TempDiffDuringHold]", enum."[UnitOfTemperature]", enum."[PerformedBy]", enum."[PerformedOn]", enum."[IsTempWithinTol]", enum."[IsTimeWithinTol]", enum."[ProcessStatus]", enum."[OverallStatus]", enum."[Result]", enum."[RawDataFilePath]", enum."[RawDataFileName]", enum."[SavedBy]"] items=["[StartRecordTime]", "[StartRecordTemp]", "[MaxRecordedTemp]", "[MaxRecordedTempTime]", "[MinRecordedTemp]", "[MinRecordedTempTime]", "[EndRecordTemp]", "[EndRecordTime]", "[RecordedMinutes]", "[StartHoldTime]", "[StartHoldTemp]", "[HoldTimeMaxTemp]", "[HoldTimeMaxTempTime]", "[HoldTimeMinTemp]", "[HoldTimeMinTempTime]", "[EndHoldTime]", "[EndHoldTemp]", "[HoldDurationMinutes]", "[TempDiffDuringHold]", "[UnitOfTemperature]", "[PerformedBy]", "[PerformedOn]", "[IsTempWithinTol]", "[IsTimeWithinTol]", "[HoldTimePercentage]", "[ProcessStatus]", "[OverallStatus]", "[SequenceStatus]", "[Parameter1]", "[Parameter2]", "[Parameter3]", "[Parameter4]", "[Parameter5]", "[Parameter6]", "[Parameter7]", "[Parameter8]", "[Parameter9]", "[Parameter10]", "[Parameter11]", "[Parameter12]", "[Result]", "[RawDataFile]", "[RawDataFilePath]", "[RawDataFileName]", "[OutputSetId]", "[SavedBy]", "[SavedOn]", "[Inactive]"] ("[TransactionResult] v02")
            w2550 = T52[] [enum."h.[ProcedureNo]", enum."h.[ProcedureRev]", enum."h.[HoldTemperature]", enum."h.[UnitOfTemperature]", enum."h.[HoldTime]", enum."h.[WPSNo]", enum."h.[ProcedureRev]"] items=["h.[TransactionNo]", "h.[ProcedureNo]", "h.[ProcedureRev]", "h.[WPSNo]", "h.[WPSRev]", "h.[HoldTemperature]", "h.[UnitOfTemperature]", "h.[HoldTime]", "h.[AdditionalProcs]", "h.[OutputSetId]", "h.[PermittedTempDiff]", "h.[PermittedTimeDiff]", "j.[Description]", "i.[itemNo]", "i.[OrderNo]", "i.[OperationNo]", "i.[Qty]", "i.[UnitOfQty]", "i.[NCRIndicator]", "i.[NCRNo]", "i.[CustomerID]", "i.[Customer]", "i.[Project]", "i.[SalesOrderNo]", "i.[SalesOrderItemNo]", "i.[MaterialNo]", "i.[MaterialDesc]", "i.[MaterialRev]", "i.[SerialNos]", "i.[Notes]", "i.[TC01]", "i.[TC02]", "i.[TC03]", "i.[TC04]", "i.[TC05]", "i.[TC06]", "i.[TC01Plot]", "i.[TC02Plot]", "i.[TC03Plot]", "i.[TC04Plot]", "i.[TC05Plot]", "i.[TC06Plot]"]
            w2530 = T52[] [enum."h.[TransactionNo]", enum."i.[itemNo]", enum."i.[OrderNo]", enum."i.[OperationNo]", enum."i.[Qty]", enum."i.[NCRNo]", enum."i.[Customer]", enum."i.[Project]", enum."i.[SalesOrderNo]", enum."i.[SalesOrderItemNo]", enum."i.[MaterialNo]", enum."i.[MaterialDesc]", enum."i.[MaterialRev]", enum."i.[SerialNos]", enum."i.[TC01]", enum."i.[TC02]", enum."i.[TC03]", enum."i.[TC04]", enum."i.[TC05]", enum."i.[TC06]", enum."i.[TC01Plot]", enum."i.[TC02Plot]", enum."i.[TC03Plot]", enum."i.[TC04Plot]", enum."i.[TC05Plot]", enum."i.[TC06Plot]", enum."i.[Notes]", enum."h.[PermittedTempDiff]", enum."h.[PermittedTimeDiff]"] items=["h.[TransactionNo]", "h.[ProcedureNo]", "h.[ProcedureRev]", "h.[WPSNo]", "h.[WPSRev]", "h.[HoldTemperature]", "h.[UnitOfTemperature]", "h.[HoldTime]", "h.[AdditionalProcs]", "h.[OutputSetId]", "h.[PermittedTempDiff]", "h.[PermittedTimeDiff]", "j.[Description]", "i.[itemNo]", "i.[OrderNo]", "i.[OperationNo]", "i.[Qty]", "i.[UnitOfQty]", "i.[NCRIndicator]", "i.[NCRNo]", "i.[CustomerID]", "i.[Customer]", "i.[Project]", "i.[SalesOrderNo]", "i.[SalesOrderItemNo]", "i.[MaterialNo]", "i.[MaterialDesc]", "i.[MaterialRev]", "i.[SerialNos]", "i.[Notes]", "i.[TC01]", "i.[TC02]", "i.[TC03]", "i.[TC04]", "i.[TC05]", "i.[TC06]", "i.[TC01Plot]", "i.[TC02Plot]", "i.[TC03Plot]", "i.[TC04Plot]", "i.[TC05Plot]", "i.[TC06Plot]"]  # h.[TransactionNo],i.[OrderNo] 2014-09-27 11:16
            w2506 = string[] ["Channel to Probe Mapping"]  # 8
            w2541 = string[] ["Furnace Serial No", "Last Inspection Date", "Next Inspection Due Date"]  # 7
            w2532 = string[] ["WPS/Ref", "WPS Rev", "Hold Temperature", "WPS Details Temperature Units", "Hold Time (HH:MM)", "Extra WPS", "Extra Rev"]  # 4
            w2545 = string[] ["Name", "Model", "Equipment Serial No.", "Last Calibration Date", "Next Calibration Date", "Equipment ID", "Notice Period", "Calibration Required"]  # 3
            w2525 = string[] ["Additional WPS Number"]  # 5
            w2546 = string[] ["Sequence Number", "Ramp Rate", "Target Temperature", "Hold Time Duration"]  # 2
            w2531 = string[] ["Transaction No", "No.", "Order No.", "Oper. No.", "Qty.", "NCR No.", "Customer Name", "Project", "Sales Order", "Item No.", "Material", "Material Description", "Revision", "Serial No.", "TC1", "TC2", "TC3", "TC4", "TC5", "TC6", "TC01Plot", "TC02Plot", "TC03Plot", "TC04Plot", "TC05Plot", "TC06Plot", "Notes", "Permitted Temp Diff", "Permitted Time Diff"]  # 1
            # "Module -> Equipment"
            # "In DB h.[AdditionalProcs] is stored as , seperated spreadsheet string\nWe want to split by \\r\\n instead of ,\nThere may also be more than 1 blank rows to cater for Retrieval \nand giving an extra empty row to MCListBox. So we need to remove when reporting."
            # "Rev removed"
            # "Rev -> WPS Rev"
            # "Skip:\n(From PartDetails MCListbox)\nUser, Customer No.,NCR Boolean\n\nAdded:\n(Not Part of Part Details MCListbox) \nPermitted Temp Diff,Permitted Time Diff"
            # "6"
            # "Don't Display Transaction No again"
            # "eg..\n[TransactionRunNo], 1\nTransaction No, 1000123\nNo. 1\nOrder No., 101"
            # "All Orders share the\nsame TransactionResult"
            # "2014-09-28\nReport (Excel)"
            # "Phase 2 has  extra [HoldTimeDuration] Column"
            # "Instead of SRTRS.Setup.ProcedureItem\nBecause we want to choose based on [TransactionRunNo"
            # "Instead of  SRTRS.Setup.Header\nBecause we want to choose based on [TransactionRunNo]"
            # "USE DB"
            n1456 = local read "Transaction (Report Buffer)"() -> (w2536:T19)
            n1457 = Unbundle By Name(w2536) -> ("TransactionNo"=w2535:string, "TransactionRunNo"=w2510:string)
            n1458 = Bundle("TransactionNo"=w2535, "TransactionRunNo"=w2510) -> (w2494:T65)  [unwired: 1 in]
            n1459 = call "DB - [Setup].[Item] (Part Details).vi"("DB - Setup Item Enum"=DB_-_Setup_Item_Enum."SELECT h.[TransactionNo], i.[OrderNo]", "DB.Schema.Table Array"=string[] ["SRTRS.Execute.Header", "SRTRS.Execute.Item", "SRTRS.MasterData.OutputSet"], "Transaction"=w2494) -> ("2D Results"=w2551:string[][], "SUMMARY"=w2552:errorcluster)  [unwired: 7 in, 4 out]
            n1460 = Delete From Array(array=w2531, index=0) -> (array with subset deleted=w2526:string[])  [unwired: 1 in, 1 out]
            n1461 = Delete From Array(array=w2530, index=0) -> (array with subset deleted=w2527:T52[])  [unwired: 1 in, 1 out]
            n1462 = Build Array "Col0\nCol1"("Transaction Run No" ("string"), w2510) -> (w2509:string[])
            n1463 = Build Array "New Row"(w2509) -> (w2499:string[][])
            n1464 = Index Array(array=w2551, index (col)=DB_-_[TransactionNo],[OrderNo]."i.[OrderNo]" ("h.[TransactionNo],i.[OrderNo]\n2014-09-27 11:16")) -> (element=w2554:string[])  [unwired: 1 in]
            n1465 = Build Array("SRTRS.Execute.ProcedureItem" ("DB.Schema.Table")) -> (w2537:string[])
            n1466 = call "DB - [Setup].[Item] (Part Details).vi"("DB - Setup Item Enum"=DB_-_Setup_Item_Enum."SELECT [Setup].[ProcedureItem]", "DB.Schema.Table Array"=w2537, "Transaction"=w2494, "error in (no error)"=w2552) -> ("2D Results"=w2544:string[][], "SUMMARY"=w2496:errorcluster)  [unwired: 6 in, 4 out]
            n1467 = Build Array (concatenate)(w2546, w2544) -> (w2543:string[][])
            n1468 = Transpose 2D Array(2D array=w2543) -> (transposed array=w2498:string[][])
            n1469 = local read "Logon"() -> (w2520:T21)
            n1470 = local read "ReportList Cluster"() -> (w2497:T18)
            n1471 = Unbundle By Name(w2520) -> ("PlantID"=w2521:string)
            n1472 = Unbundle By Name(w2497) -> ("[IsManual]"=w2493:string)
            n1473 = case shown="\"1\"" w2493 {
              tunnel: w2496 -> [w2559 w2581]
              tunnel: [w2560 w2577] -> w2495
              tunnel: [w2559 w2567] -> w2488
              tunnel: w2494 -> [_ w2572]
              tunnel: [w2558 w2571] -> w2491
              tunnel: [w2556 w2565] -> w2489
              frame "0", Default {
                n1474 = property on="Channel to Probe Mapping" class="Clust (strict)"() -> ("Value"=w2557:cluster{"Channel to Probe Mapping":string})  [unwired: 2 in, 2 out]
                n1475 = property on="Equipment Details" class="MCListbox (strict)"() -> ("ItemNames"=w2560:string[][])  [unwired: 2 in, 2 out]
                n1476 = Unbundle By Name(w2557) -> ("Channel to Probe Mapping"=w2556:string)
                n1477 = property on="Furnace Details" class="Clust (strict)"() -> ("Value"=w2558:T6)  [unwired: 2 in, 2 out]
              }
              frame "1" {
                w2564 = 1  # Channel Mapping
                # "IsManual"
                n1478 = call "DB - [Setup].[Item] (Part Details).vi"("DB - Setup Item Enum"=DB_-_Setup_Item_Enum."SELECT [EquipmentxId]", "DB.Schema.Table Array"=string[] ["SRTRS.Execute.Header"], "Transaction"=w2572, "error in (no error)"=w2581) -> ("1D Results"=w2574:string[], "SUMMARY"=w2575:errorcluster)  [unwired: 6 in, 4 out]
                n1479 = Index Array(array=w2574) -> (element #1=w2570:string, element #2=w2569:string, element #3=w2573:string)  [unwired: 3 in]
                n1480 = local read "Date Format (UserDefined)"() -> (w2583:string)
                n1481 = local read "Logon"() -> (w2582:T21)
                n1482 = Unbundle By Name(w2582) -> ("LanguageID"=w2576:string)
                n1483 = call "DB - [Config].[System].vi"("DB Connection"=T53 {"Open"=TRUE, "Close"=FALSE}, "[LanguageId]"=w2576, "Date Format (User Defined)"=w2583, "AND IN (EquipmentIDx,..)"=TRUE, "error in (no error)"=w2575, "[PlantId]"=w2570, "[SystemId]"=w2569, "<Values>"=w2573) -> ("connection reference"=w2561:T66, "Furnace Details"=w2571:T6, "Equipment Details (Itemnames)"=w2577:string[][], "SUMMARY"=w2568:errorcluster)  [unwired: 4 in]
                n1484 = call "DB - [Config].[Controller].vi"("[SystemId]"=w2569, "[PlantId]"=w2570, "DB Connection"=T53 {"Open"=FALSE, "Close"=TRUE}, "error in (no error)"=w2568, "connection reference"=w2561) -> ("SUMMARY"=w2567:errorcluster, "data"=w2566:string[])  [unwired: 4 in, 1 out]
                n1485 = Index Array(array=w2566, index=w2564) -> (element=w2565:string)
              }
            }
            n1486 = Build Array (concatenate)(w2545, w2495) -> (w2542:string[][])
            n1487 = Transpose 2D Array(2D array=w2542) -> (transposed array=w2507:string[][])
            n1488 = Cluster To Array(cluster=w2491) -> (array=w2492:string[])
            n1489 = Build Array(w2541, w2492) -> (w2490:string[][])
            n1490 = Transpose 2D Array(2D array=w2490) -> (transposed array=w2508:string[][])
            n1491 = local read "Logon Extra"() -> (w2514:T25)
            n1492 = Unbundle By Name(w2514) -> ("UserName"=w2502:string)
            n1493 = Build Array (concatenate) "Col0\nCol1"(w2506, w2489) -> (w2505:string[])
            n1494 = Build Array "Col0\nCol1"("Username" ("string"), w2502) -> (w2501:string[])
            n1495 = call "DB - [Execute].[Transaction].vi"("DB.Schema.Table"="SRTRS.Execute.TransactionResult", "Transaction"=w2494, "DB - Execute Transaction"=DB_-_Execute_Transaction_Enum."SELECT [TransactionResult]", "[TransactionResult] v02"=w2540) -> ("1D Results"=w2534:string[], "SUMMARY"=w2533:errorcluster)  [unwired: 12 in, 2 out]
            n1496 = for {
              tunnel: w2513 -> [w2585] mode=indexing
              tunnel: [w2584] -> w2512 mode=indexing
              n1497 = Format Into String(w2585) -> (resulting string=w2584:string)  [unwired: 3 in, 1 out]
            }
            n1498 = for {
              tunnel: w2540 -> [w2592] mode=indexing
              tunnel: w2534 -> [w2587] mode=indexing
              tunnel: [w2591] -> w2504 mode=indexing
              tunnel: w2512 -> [w2590]
              n1499 = Format Into String(w2592) -> (resulting string=w2589:string)  [unwired: 3 in, 1 out]
              n1500 = Search 1D Array(1D array=w2590, element=w2589) -> (index of element=w2588:i32)  [unwired: 1 in]
              n1501 = case shown="0, Default" w2588 {
                tunnel: w2587 -> [w2595 w2596]
                tunnel: [w2593 w2596] -> w2586
                frame 0, Default {
                  # "Double Convert\nBit Type"
                  n1502 = call "DB - Convert BIT Type.vi"("BIT Type (eg Inactive)"=w2595) -> ("Boolean"=w2594:bool)  [unwired: 2 in, 2 out]
                  n1503 = call "DB - Convert BIT Type.vi"("Boolean"=w2594) -> ("BIT (eg Inactive)"=w2593:string)  [unwired: 2 in, 2 out]
                }
                frame -1 {
                }
              }
              n1504 = Build Array(w2589, w2586) -> (w2591:string[])
            }
            n1505 = for {
              tunnel: w2551 -> [w2617] mode=indexing
              tunnel: w2527 -> [w2624]
              tunnel: w2498 -> [w2614]
